vi "Find All SLSC Switch Custom Devices.vi"(8 "error in (no error)":errorcluster, 11 "Target in":refnum<k24>) -> (0 "error out":errorcluster, 2 "SLSC Switch Custom Device Ref IDs":T1[](array[typedef]) format="%.0x", 3 "Target out":refnum<k24>)   [LabVIEW 2017, in "SLSC Switch Scripting.lvlib"]
uses:
  SLSC Switch Scripting.lvlib
  NationalInstruments.VeriStand.SystemDefinitionAPI
  <vilib>/NI Veristand/Custom Device API/Custom Device Item Ref.ctl
  SLSC Scripting Constants.vi
  <vilib>/NI VeriStand/Custom Device API/Custom Device API.lvlib
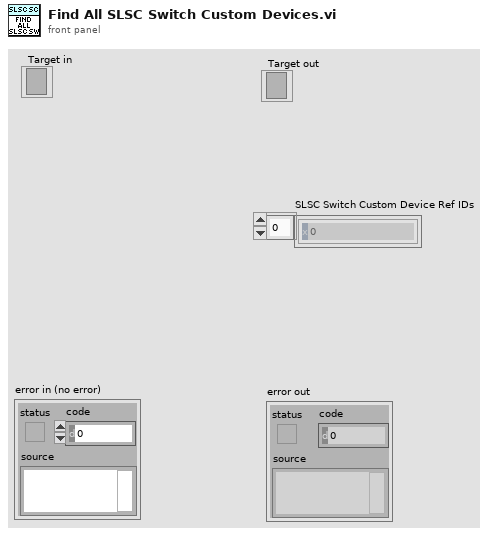
[diagram p1: front panel]
types:
  T1 = typedef "Custom Device API.lvlib/Custom Device Item Ref.ctl" = u64
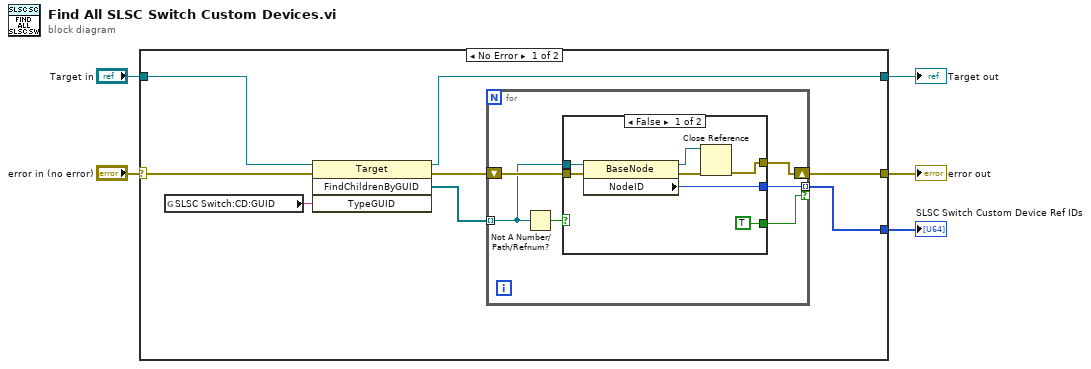
[diagram p0: block diagram]
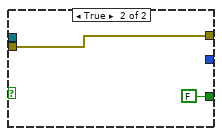
[diagram p2: hidden frame]
diagram:
  n1 = case shown="No Error" "error in (no error)" {
    selector: "error in (no error)" -> [w13 w30]
    tunnel: [w7 w30] -> w2
    tunnel: "Target in" -> [w12 w29]
    tunnel: [w9 w29] -> w3
    tunnel: [w8 _] -> w1
    frame No Error {
      n2 = global read "SLSC Scripting Constants.vi" "SLSC Switch:CD:GUID"() -> (w6:string)
      n3 = invoke class="Target" method="FindChildrenByGUID"(reference=w12, error in=w13, "TypeGUID"=w6) -> (reference out=w9:refnum<k24>, error out=w11:errorcluster, "FindChildrenByGUID"=w10:refnum<k24>[])  [unwired: 1 in, 1 out]
      n4 = for {
        tunnel: [w18] -> w8 mode=indexing if=w15
        tunnel: w10 -> [w16] mode=indexing
        shift-right: [w14] -> w7
        shift-left: w11 -> [w19]
        n5 = Not A Number/Path/Refnum?(number/path/refnum=w16) -> (NaN/Path/Refnum?=w17:bool)
        n6 = case shown="False" w17 {
          tunnel: w19 -> [w25 w27]
          tunnel: [w26 _] -> w18
          tunnel: w16 -> [w24 _]
          tunnel: [TRUE FALSE] -> w15
          tunnel: [w22 w27] -> w14
          frame False {
            n7 = property class="BaseNode"(reference=w24, error in=w25) -> (reference out=w20:refnum<k24>, error out=w21:errorcluster, "NodeID"=w26:u64)
            n8 = Close Reference(reference=w20, error in (no error)=w21) -> (error out=w22:errorcluster)
          }
          frame True {
          }
        }
      }
    }
    frame Error {
    }
  }
  "Target out" <- w3
  "error out" <- w2
  "SLSC Switch Custom Device Ref IDs" <- w1
